vi "Stop.vi"(8 "error in (no error)":errorcluster, 11 "TCP Comm":T1) -> (0 "error out":errorcluster)   [LabVIEW 2020, in "TCP Comms.lvlib"]
uses:
  TCP Comms.lvlib
  TCP Comm.ctl
  Ref Data.ctl
  State.ctl
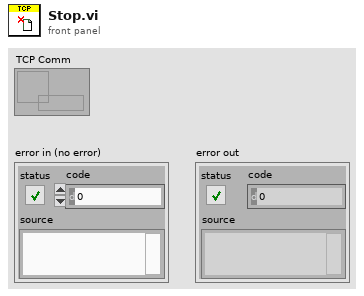
[diagram p1: front panel]
types:
  T1 = typedef "TCP Comms.lvlib/TCP Comm.ctl" = refnum<data-value>
  T2 = typedef "TCP Comms.lvlib/Ref Data.ctl" = cluster{"TCP":refnum<k5>, "State":T3, "Server":bool, "Host":string, "Port":u16, "Listener":refnum<k5>, "Start":bool, "Disconnect":bool, "TCP Valid":bool, "TLS Enabled":bool, "Immutable TLS":refnum<k36>, "Certificate DN":string}
  T3 = typedef "TCP Comms.lvlib/State.ctl" = enum16{"Idle", "Starting", "Connecting", "Connected", "Disconnecting", "Stopped"}
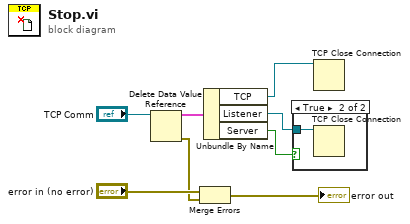
[diagram p0: block diagram]
diagram:
  n1 = Delete Data Value Reference(data value reference="TCP Comm") -> (data value=w7:T2, error out=w2:errorcluster)  [unwired: 1 in]
  n2 = Merge Errors("error in (no error)", w2) -> (→"error out":errorcluster)
  n3 = Unbundle By Name(w7) -> ("TCP"=w6:refnum<k5>, "Listener"=w4:refnum<k5>, "Server"=w5:bool)
  n4 = case shown="True" w5 {
    tunnel: w4 -> [_ w9]
    frame False {
    }
    frame True {
      n5 = TCP Close Connection(connection ID=w9) -> ()  [unwired: 2 in, 2 out]
    }
  }
  n6 = TCP Close Connection(connection ID=w6) -> ()  [unwired: 2 in, 2 out]
